vi "json From Variant.vi"(8 "error in (no error)":errorcluster, 9 "Variant":variant, 10 "path":string, 11 "JSON Document in":refnum<class "JSON Document.lvclass">) -> (0 "error out":errorcluster, 3 "JSON Document out":refnum<class "JSON Document.lvclass">)   [LabVIEW 2015, in "JSON Document.lvclass"]
uses:
  JSON Document.lvclass
  json insert/poly instances/json Insert I32 - string path.vi
  json insert/poly instances/json Insert I64 - string path.vi
  json insert/poly instances/json Insert U32 - string path.vi
  json insert/poly instances/json Insert U64 - string path.vi
  json insert/poly instances/json Insert Float - string path.vi
  json insert/poly instances/json Insert Double - string path.vi
  json insert/poly instances/json Insert Boolean - string path.vi
  json insert/poly instances/json Insert String - string path.vi
  json insert/poly instances/json Insert Path - string path.vi
  <vilib>/Utility/Data Type/NI_Data Type.lvlib
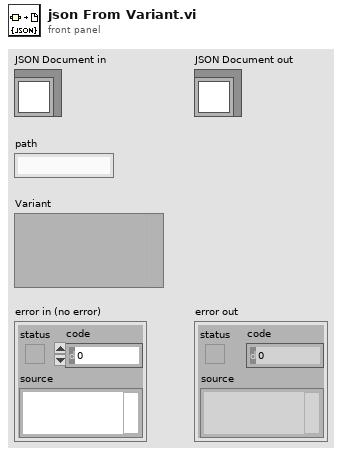
[diagram p1: front panel]
types:
  T1 = typedef "NI_Data Type.lvlib/Data Type.ctl" = enum8{"Invalid Type", "Void", "I8", "I16", "I32", "I64", "U8", "U16", "U32", "U64", "Single Float", "Double Float", "Extended Float", "Single Complex", "Double Complex", "Extended Complex", "Enum U8", "Enum U16", "Enum U32", "Enum U64", "Single Float With Unit", "Double Float With Unit", "Extended Float With Unit", "Single Complex with Unit", "Double Complex with Unit", "Extended Complex with Unit", "Boolean", "String", "Path", "Picture", "Tag", "Array", "Cluster", "Variant", "LV Variant", "Waveform", "Timestamp", "Digital Waveform", "Digital Data", "ExpressData", "Refnum", "External Data", "VI", "Poly VI", "LabVIEW Class Instance", "Fixed Point"}
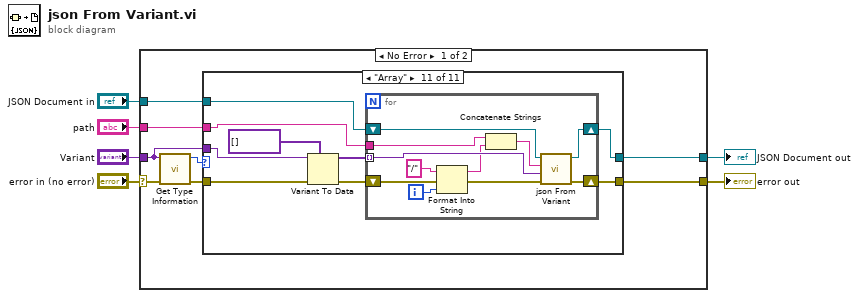
[diagram p0: block diagram]
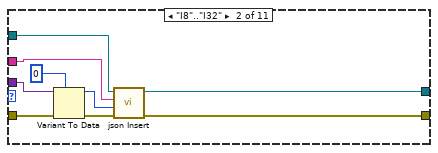
[diagram p3: hidden frame]
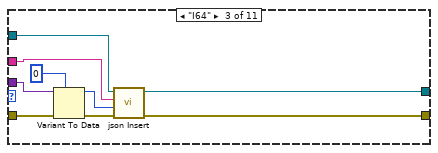
[diagram p4: hidden frame]
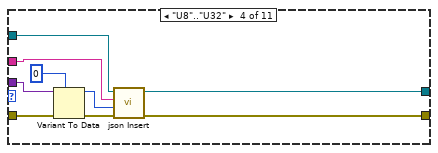
[diagram p5: hidden frame]
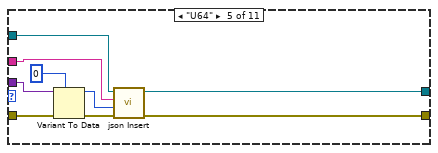
[diagram p6: hidden frame]
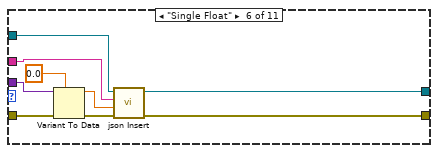
[diagram p7: hidden frame]
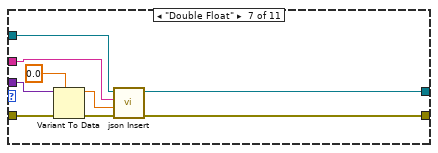
[diagram p8: hidden frame]
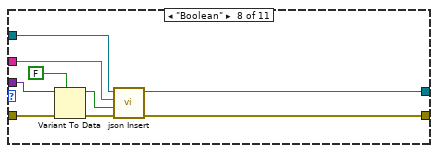
[diagram p9: hidden frame]
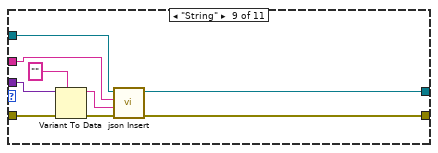
[diagram p10: hidden frame]
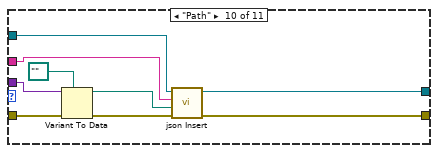
[diagram p11: hidden frame]
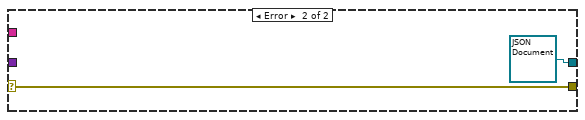
[diagram p12: hidden frame]
diagram:
  n1 = case shown="No Error" "error in (no error)" {
    selector: "error in (no error)" -> [w10 w118]
    tunnel: "Variant" -> [w13 _]
    tunnel: [w11 refnum<class "JSON Document.lvclass"> refnum ("JSON Document out")] -> w4
    tunnel: [w9 w118] -> w3
    tunnel: "JSON Document in" -> [w8 _]
    tunnel: "path" -> [w7 _]
    frame No Error {
      n2 = call <vilib>:"Get Type Information.vi"("error in (no error)"=w10, "Variant"=w13) -> ("error out"=w12:errorcluster, "Type"=w14:T1)  [unwired: 5 in, 3 out]
      n3 = case shown="\"Array\"" w14 {
        tunnel: w13 -> [_ w24 w33 w42 w51 w60 w69 w78 w87 w96 w105]
        tunnel: w12 -> [w16 w23 w32 w41 w50 w59 w68 w77 w86 w95 w104]
        tunnel: w8 -> [w15 w21 w30 w39 w48 w57 w66 w75 w84 w93 w102]
        tunnel: [w15 w19 w28 w37 w46 w55 w64 w73 w82 w91 w100] -> w11
        tunnel: [w16 w18 w27 w36 w45 w54 w63 w72 w81 w90 w99] -> w9
        tunnel: w7 -> [_ w17 w26 w35 w44 w53 w62 w71 w80 w89 w98]
        frame "Invalid Type", Default {
        }
        frame "I8".."I32" {
          n4 = Variant To Data(error in=w23, type=0, Variant=w24) -> (data=w20:i32, error out=w22:errorcluster)
          n5 = call-poly "json Insert.vi"("error in (no error)"=w22, "anything"=w20, "path"=w17, "JSON Document in"=w21) -> ("error out"=w18:errorcluster, "JSON Document out"=w19:refnum<class "JSON Document.lvclass">)  [unwired: 5 in, 1 out]
        }
        frame "I64" {
          n6 = Variant To Data(error in=w32, type=i64 0, Variant=w33) -> (data=w29:i64, error out=w31:errorcluster)
          n7 = call-poly "json Insert.vi"("error in (no error)"=w31, "anything"=w29, "path"=w26, "JSON Document in"=w30) -> ("error out"=w27:errorcluster, "JSON Document out"=w28:refnum<class "JSON Document.lvclass">)  [unwired: 5 in, 1 out]
        }
        frame "U8".."U32" {
          n8 = Variant To Data(error in=w41, type=u32 0, Variant=w42) -> (data=w38:u32, error out=w40:errorcluster)
          n9 = call-poly "json Insert.vi"("error in (no error)"=w40, "anything"=w38, "path"=w35, "JSON Document in"=w39) -> ("error out"=w36:errorcluster, "JSON Document out"=w37:refnum<class "JSON Document.lvclass">)  [unwired: 5 in, 1 out]
        }
        frame "U64" {
          n10 = Variant To Data(error in=w50, type=u64 0, Variant=w51) -> (data=w47:u64, error out=w49:errorcluster)
          n11 = call-poly "json Insert.vi"("error in (no error)"=w49, "anything"=w47, "path"=w44, "JSON Document in"=w48) -> ("error out"=w45:errorcluster, "JSON Document out"=w46:refnum<class "JSON Document.lvclass">)  [unwired: 5 in, 1 out]
        }
        frame "Single Float" {
          n12 = Variant To Data(error in=w59, type=sgl 0.0, Variant=w60) -> (data=w56:sgl, error out=w58:errorcluster)
          n13 = call-poly "json Insert.vi"("error in (no error)"=w58, "anything"=w56, "path"=w53, "JSON Document in"=w57) -> ("error out"=w54:errorcluster, "JSON Document out"=w55:refnum<class "JSON Document.lvclass">)  [unwired: 5 in, 1 out]
        }
        frame "Double Float" {
          n14 = Variant To Data(error in=w68, type=0.0, Variant=w69) -> (data=w65:dbl, error out=w67:errorcluster)
          n15 = call-poly "json Insert.vi"("error in (no error)"=w67, "anything"=w65, "path"=w62, "JSON Document in"=w66) -> ("error out"=w63:errorcluster, "JSON Document out"=w64:refnum<class "JSON Document.lvclass">)  [unwired: 5 in, 1 out]
        }
        frame "Boolean" {
          n16 = Variant To Data(error in=w77, type=FALSE, Variant=w78) -> (data=w74:bool, error out=w76:errorcluster)
          n17 = call-poly "json Insert.vi"("error in (no error)"=w76, "anything"=w74, "path"=w71, "JSON Document in"=w75) -> ("error out"=w72:errorcluster, "JSON Document out"=w73:refnum<class "JSON Document.lvclass">)  [unwired: 5 in, 1 out]
        }
        frame "String" {
          n18 = Variant To Data(error in=w86, type="", Variant=w87) -> (data=w83:string, error out=w85:errorcluster)
          n19 = call-poly "json Insert.vi"("error in (no error)"=w85, "anything"=w83, "path"=w80, "JSON Document in"=w84) -> ("error out"=w81:errorcluster, "JSON Document out"=w82:refnum<class "JSON Document.lvclass">)  [unwired: 5 in, 1 out]
        }
        frame "Path" {
          n20 = Variant To Data(error in=w95, type=path "", Variant=w96) -> (data=w92:path, error out=w94:errorcluster)
          n21 = call-poly "json Insert.vi"("error in (no error)"=w94, "anything"=w92, "path"=w89, "JSON Document in"=w93) -> ("error out"=w90:errorcluster, "JSON Document out"=w91:refnum<class "JSON Document.lvclass">)  [unwired: 5 in, 1 out]
        }
        frame "Array" {
          n22 = Variant To Data(error in=w104, type=variant[] [], Variant=w105) -> (data=w101:variant[], error out=w103:errorcluster)
          n23 = for {
            tunnel: w101 -> [w114] mode=indexing
            shift-right: [w116] -> w99
            shift-left: w103 -> [w108]
            shift-right: [w117] -> w100
            shift-left: w102 -> [w115]
            tunnel: w98 -> [w111]
            i -> [w113]
            n24 = Format Into String(initial string="/", error in=w108, w113) -> (resulting string=w110:string, error out=w107:errorcluster)  [unwired: 1 in]
            n25 = Concatenate Strings(w111, w110) -> (w109:string)
            n26 = call "json From Variant.vi"("error in (no error)"=w107, "Variant"=w114, "path"=w109, "JSON Document in"=w115) -> ("error out"=w116:errorcluster, "JSON Document out"=w117:refnum<class "JSON Document.lvclass">)  [unwired: 6 in]
          }
        }
      }
    }
    frame Error {
    }
  }
  "error out" <- w3
  "JSON Document out" <- w4
